vi "Set Open Weather Session.vi"(8 "Error In":errorcluster, 10 "Open Weather Session":refnum<class "Open Weather Session.lvclass">, 11 "Dashboard In":refnum<class "Dashboard.lvclass">) -> (0 "Error Out":errorcluster, 3 "Dashboard Out":refnum<class "Dashboard.lvclass">)   [LabVIEW 2021, in "Dashboard.lvclass"]
uses:
  Dashboard.lvclass
  <vilib>/Memosfet/OpenWeatherAPI/Open Weather Session/Open Weather Session.lvclass
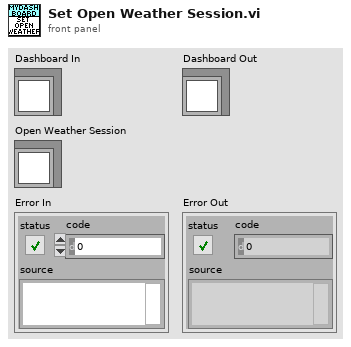
[diagram p1: front panel]
types:
  T1 = typedef "Dashboard.lvclass/Data.ctl" = cluster{"Central Message Handler":refnum<class "Central Message Handler.lvclass">, "Display":refnum<class "Display.lvclass">, "FPGA Reference":T2, "Open Weather Session":refnum<class "Open Weather Session.lvclass">, "Processes":T3}
  T2 = typedef "Dashboard.lvclass/FPGA Reference.ctl" = refnum<k20>
  T3 = typedef "Dashboard.lvclass/Processes.ctl" = cluster{"Display Manager":refnum<class "Display Manager.lvclass">, "Audio Analyzer":refnum<class "Audio Analyzer.lvclass">, "Draw Frame":refnum<class "Draw Frame.lvclass">, "Error Handling":refnum<class "Error Handling.lvclass">, "Sequencer":refnum<class "Sequencer.lvclass">}
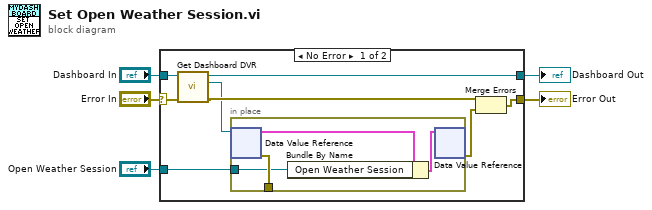
[diagram p0: block diagram]
diagram:
  n1 = case shown="No Error" "Error In" {
    selector: "Error In" -> [w10 w18]
    tunnel: [w12 w18] -> w2
    tunnel: [w9 w19] -> w5
    tunnel: "Dashboard In" -> [w11 w19]
    tunnel: "Open Weather Session" -> [w6 _]
    frame No Error {
      n2 = call "Get Dashboard DVR.vi"("Error In"=w10, "Dashboard In"=w11) -> ("Error Out"=w8:errorcluster, "DVR"=w7:refnum<data-value>, "Dashboard Out"=w9:refnum<class "Dashboard.lvclass">)  [unwired: 7 in]
      n3 = in-place {
        in-place-border: [w17] -> _
        in-place-border: w6 -> [w14]
        n4 = in-place-dvr #1(w7) -> (w16:T1, w17:errorcluster)
        n5 = Bundle By Name(cluster=w16, "Open Weather Session"=w14) -> (w15:T1)
        n6 = in-place-dvr #1(w15) -> (w13:errorcluster)  [unwired: 1 out]
      }
      n7 = Merge Errors(w8, w13) -> (w12:errorcluster)
    }
    frame Error {
    }
  }
  "Dashboard Out" <- w5
  "Error Out" <- w2
